vi "Laboratory_practice7.vi"() -> ()   [LabVIEW 2022 SP3]
panel:
  out "Peak to Peak":dbl
  in  "stop":bool
  out "RMS":dbl
  out "Waveform Graph":dynamicdata(graph)
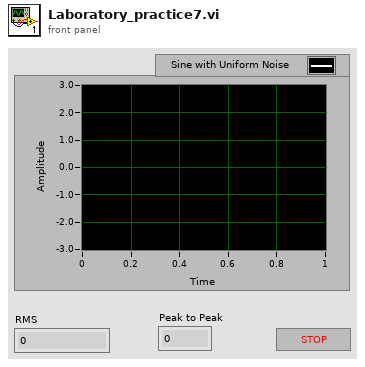
[diagram p1: front panel]
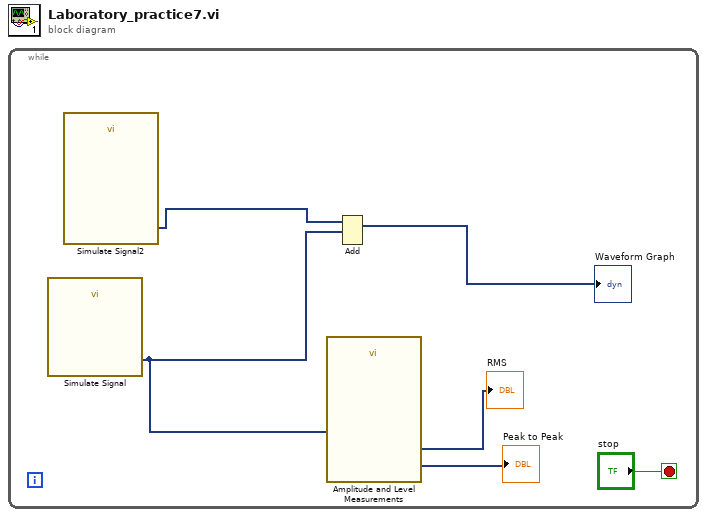
[diagram p0: block diagram]
diagram:
  n1 = while {
    stop <- "stop" stop-if-true
    n2 = call "Simulate Signal"() -> ("Sine"=w3:dynamicdata)  [unwired: 14 in, 1 out]
    n3 = call "Simulate Signal2"() -> ("Sine with Uniform Noise"=w2:dynamicdata)  [unwired: 14 in, 1 out]
    n4 = call "Amplitude and Level Measurements"("Signals"=w3) -> ("RMS"=→"RMS":dynamicdata, "Peak to Peak"=→"Peak to Peak":dynamicdata)  [unwired: 12 in, 1 out]
    n5 = Add(1:w3, 2:w2) -> (0:→"Waveform Graph":dynamicdata)  [unwired: 1 in, 1 out]
  }
